vi "Cast Command to Transfer Group.vi"(8 "error in (no error)":errorcluster, 10 "command parameters":T1, 11 "Plugin Thread in":refnum<class "Plugin Thread.lvclass">) -> (0 "error out":errorcluster, 1 "Transfer Group iteration":u64, 2 "Transfer Group id":u8, 3 "Plugin Thread out":refnum<class "Plugin Thread.lvclass">, 5 "Transfer Group late count":i32)   [LabVIEW 2019, in "DSF Core.lvlib" / "Plugin Thread.lvclass"]
uses:
  Thread/Plugin/Plugin Thread.lvclass
  Interface/Plugin/Command Parameters.ctl
  Thread/Plugin/Plugin Thread.lvclass/Plugin Thread.ctl
  Interface/Plugin/Plugin Interface.lvclass
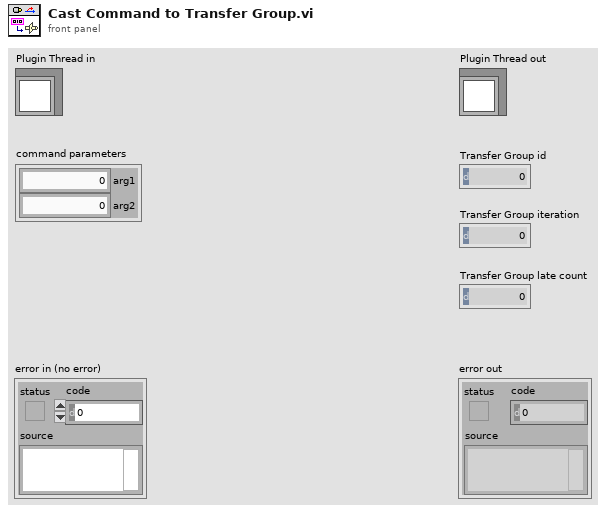
[diagram p1: front panel]
types:
  T1 = typedef "DSF Core.lvlib/Plugin Interface.lvclass/Command Parameters.ctl" = cluster{"arg1":u64, "arg2":u64}
  T2 = cluster{"Transfer Group ID":i32, "Transfer Group Late Count":i32, "Transfer Group Iteration":u64}
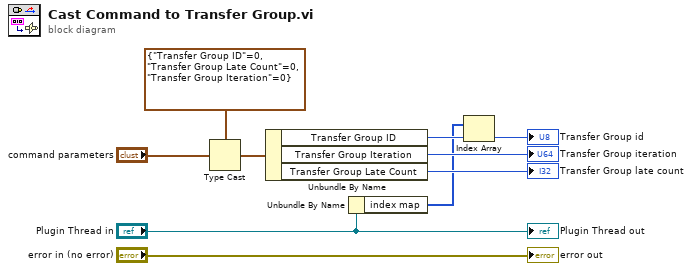
[diagram p0: block diagram]
diagram:
  n1 = Type Cast(type=T2 {"Transfer Group ID"=0, "Transfer Group Late Count"=0, "Transfer Group Iteration"=0}, x="command parameters") -> (*(type *) &x=w9:T2)
  n2 = Unbundle By Name(w9) -> ("Transfer Group ID"=w3:i32, "Transfer Group Iteration"=→"Transfer Group iteration":u64, "Transfer Group Late Count"=→"Transfer Group late count":i32)
  n3 = Unbundle By Name("Plugin Thread in") -> ("index map"=w1:u8[])
  n4 = Index Array(array=w1, index=w3) -> (element=→"Transfer Group id":u8)
  "error out" <- "error in (no error)"
  "Plugin Thread out" <- "Plugin Thread in"
